vi "AlliGator Remove Duplicate Fit Result Constraint.vi"(8 "error in (no error)":errorcluster, 9 "ArrayElt":T1, 11 "NewArray in":T1[](array[typedef])) -> (0 "error out":errorcluster, 3 "NewArray out":T1[](array[typedef]))   [LabVIEW 2021, in "AlliGator Decay Fit Parameter Map.lvlib"]
uses:
  AlliGator Decay Fit Parameter Map.lvlib
  <userlib>/_OpenG.lib/array/array.llb/openg_array.lvlib
  <userlib>/_OpenG.lib/array/array.llb/Search 1D Array (I16)__ogtk.vi
  Fits/IRF(X)PSED/Decay Fit Result Constraint.ctl
  Fits/Fits.lvlib
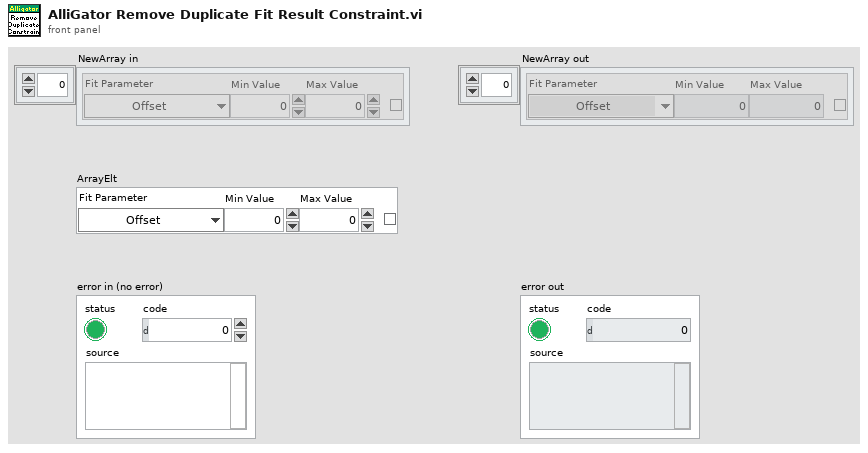
[diagram p1: front panel]
types:
  T1 = typedef "Fits.lvlib/Decay Fit Result Constraint.ctl" = cluster{"Fit Parameter":enum16{"Offset", "Baseline", "A_1", "tau_1", "A_2", "tau_2", "<tau>_a", "f1_a", "f2_a", "<tau>_i", "f1_i", "f2_i", "-", "R^2", "Chi^2", "Max Relative Residual", "<Residual ACF>", "Residual ACF SDV", "tau_2/tau_1"}, "Min Value":dbl, "Max Value":dbl, "Use Constraint":bool}
  T2 = enum16{"Offset", "Baseline", "A_1", "tau_1", "A_2", "tau_2", "<tau>_a", "f1_a", "f2_a", "<tau>_i", "f1_i", "f2_i", "-", "R^2", "Chi^2", "Max Relative Residual", "<Residual ACF>", "Residual ACF SDV", "tau_2/tau_1"}
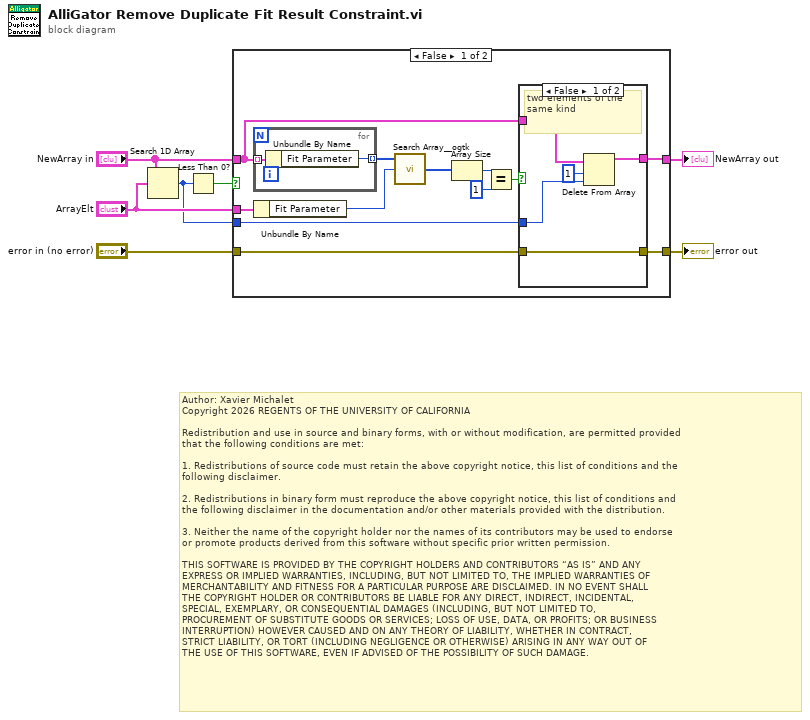
[diagram p0: block diagram]
diagram:
  # "Author: Xavier Michalet\nCopyright 2026 REGENTS OF THE UNIVERSITY OF CALIFORNIA\n\nRedistribution and use in source and binary forms, with or without modification, are permitted provided\nthat the following conditions are met:\n\n1. Redistributions of source code must retain the above copyright notice, this list of conditions and the\nfollowing disclaimer.\n\n2. Redistributions in binary form must reproduce the above copyright notice, this list of conditions and\nthe following disclaimer in the documentation and/or other materials provided with the distribution.\n\n3. Neither the name of the copyright holder nor the names of its contributors may be used to endorse \nor promote products derived from this software without specific prior written permission.\n\nTHIS SOFTWARE IS PROVIDED BY THE COPYRIGHT HOLDERS AND CONTRIBUTORS “AS IS” AND ANY \nEXPRESS OR IMPLIED WARRANTIES, INCLUDING, BUT NOT LIMITED TO, THE IMPLIED WARRANTIES OF\nMERCHANTABILITY AND FITNESS FOR A PARTICULAR PURPOSE ARE DISCLAIMED. IN NO EVENT SHALL\nTHE COPYRIGHT HOLDER OR CONTRIBUTORS BE LIABLE FOR ANY DIRECT, INDIRECT, INCIDENTAL, \nSPECIAL, EXEMPLARY, OR CONSEQUENTIAL DAMAGES (INCLUDING, BUT NOT LIMITED TO, \nPROCUREMENT OF SUBSTITUTE GOODS OR SERVICES; LOSS OF USE, DATA, OR PROFITS; OR BUSINESS\nINTERRUPTION) HOWEVER CAUSED AND ON ANY THEORY OF LIABILITY, WHETHER IN CONTRACT, \nSTRICT LIABILITY, OR TORT (INCLUDING NEGLIGENCE OR OTHERWISE) ARISING IN ANY WAY OUT OF\nTHE USE OF THIS SOFTWARE, EVEN IF ADVISED OF THE POSSIBILITY OF SUCH DAMAGE."
  n1 = Search 1D Array(1D array="NewArray in", element="ArrayElt") -> (index of element=w1:i32)  [unwired: 1 in]
  n2 = Less Than 0?(x=w1) -> (x < 0?=w6:bool)
  n3 = case shown="False" w6 {
    tunnel: "NewArray in" -> [w10 w29]
    tunnel: "error in (no error)" -> [w13 w30]
    tunnel: [w12 w30] -> w4
    tunnel: [w9 w29] -> w3
    tunnel: "ArrayElt" -> [w19 _]
    tunnel: w1 -> [w8 _]
    frame False {
      n4 = for {
        tunnel: w10 -> [w28] mode=indexing
        tunnel: [w27] -> w18 mode=indexing
        n5 = Unbundle By Name(w28) -> ("Fit Parameter"=w27:T2)
      }
      n6 = Unbundle By Name(w19) -> ("Fit Parameter"=w17:T2)
      n7 = call-poly <userlib>:"Search Array__ogtk.vi"("Array"=w18, "Element Data"=w17) -> ("Indices of Elements"=w16:i32[])  [unwired: 7 in]
      n8 = Array Size(array=w16) -> (size(s)=w15:i32)
      n9 = Equal?(x=w15, y=1) -> (x = y?=w11:bool)
      n10 = case shown="False" w11 {
        tunnel: w13 -> [w20 w26]
        tunnel: [w20 w26] -> w12
        tunnel: w10 -> [w24 w25]
        tunnel: [w23 w25] -> w9
        tunnel: w8 -> [w22 _]
        frame False {
          # "two elements of the same kind"
          n11 = Delete From Array(array=w24, length=1, index=w22) -> (array with subset deleted=w23:T1[])  [unwired: 1 out]
        }
        frame True {
        }
      }
    }
    frame True {
      # "Unexpected situation: ignore"
    }
  }
  "error out" <- w4
  "NewArray out" <- w3
